vi "Record_to_TDMS.vi"() -> ()   [LabVIEW 2019]
uses:
  SubVIs/TypeDefs/StateRecording.ctl
  <vilib>/DAQmx/read.llb/DAQmx Read (Analog 1D Wfm NChan NSamp).vi
  <vilib>/DAQmx/create/channels.llb/DAQmx Create Channel (AI-Voltage-Basic).vi
  <vilib>/DAQmx/configure/timing.llb/DAQmx Timing (Sample Clock).vi
  <vilib>/DAQmx/miscellaneous.llb/DAQmx Fill In Error Info.vi
  <vilib>/measure/madcrms.llb/Basic Averaged DC-RMS for 1 Chan.vi
  <vilib>/express/express analysis/Spectral/Block/exnSpectralBlock spectral measurements RMS poly.vi
  <vilib>/express/express analysis/Spectral/Block/exnSpectralBlock spectral measurements RMS WFM.vi
  <vilib>/express/express analysis/Spectral/XNode/ExpressSpectralMeasurementsBlockNode.xnode
  <vilib>/measure/NI_MAPro.lvlib
panel:
  out "Elapsed Time (s)":dbl
  in  "stop":bool
  in  "Pause time [s]":dbl=15.0 caption="Time Target (s)"
  out "State":string
  in  "Record":bool
  out "Waveform":waveform(dbl)[](graph)
  out "Spectrum":cluster{"f0":dbl, "df":dbl, "magnitude":dbl[]}(graph)
  in  "sample rate":dbl=10000.0 format="%#_13g"
  in  "samples per channel":i32=10000
  in  "Filename":string
  in  "Recording time [s]":dbl=15.0 caption="Time Target (s)"
  in  "Number of recordings":i32
  in  "Recording directory":path
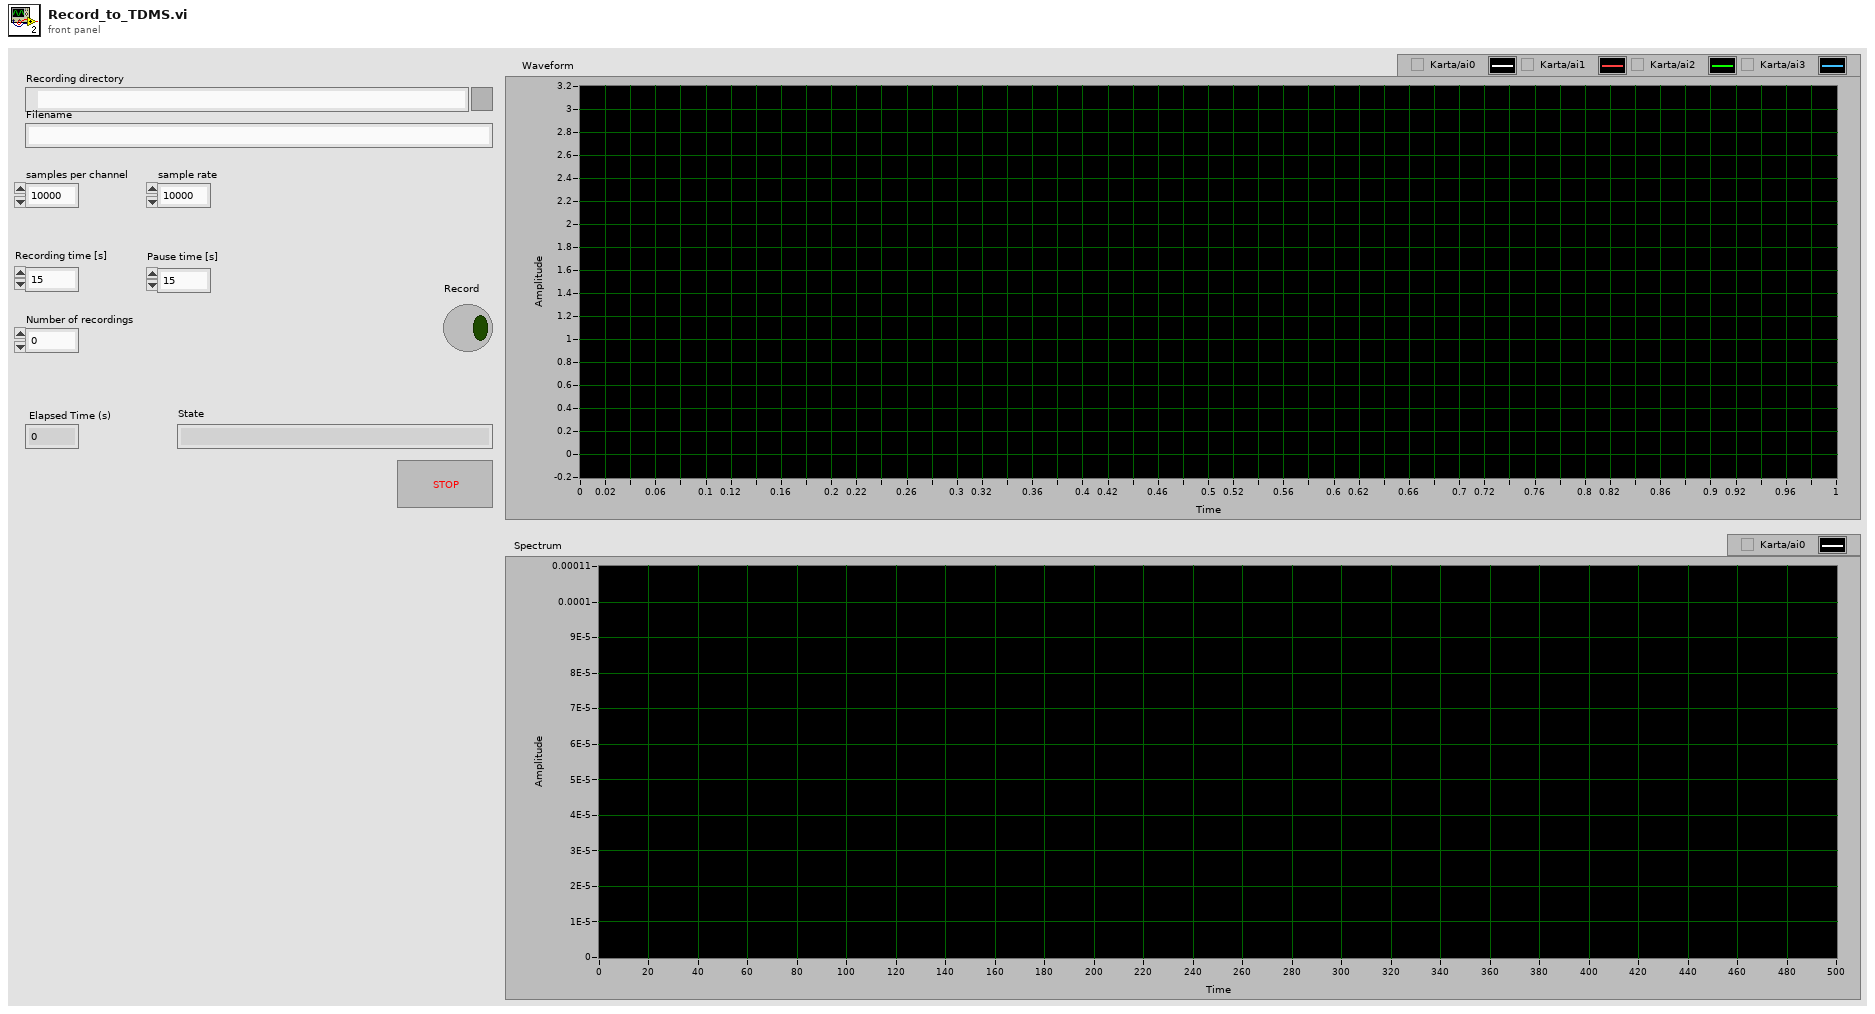
[diagram p1: front panel]
types:
  T1 = typedef "StateRecording.ctl" = enum16{"IDLE", "RECORDING", "PAUSE"}
  T2 = enum16{"open", "open or create", "create or replace", "create", "open (read-only)"}
  T3 = cluster{"averaging mode":u16, "weighting mode":u16, "number of averages":u32}
  T4 = cluster{"dB On (F)":bool, "unwrap phase (F)":bool, "convert to degree (F)":bool}
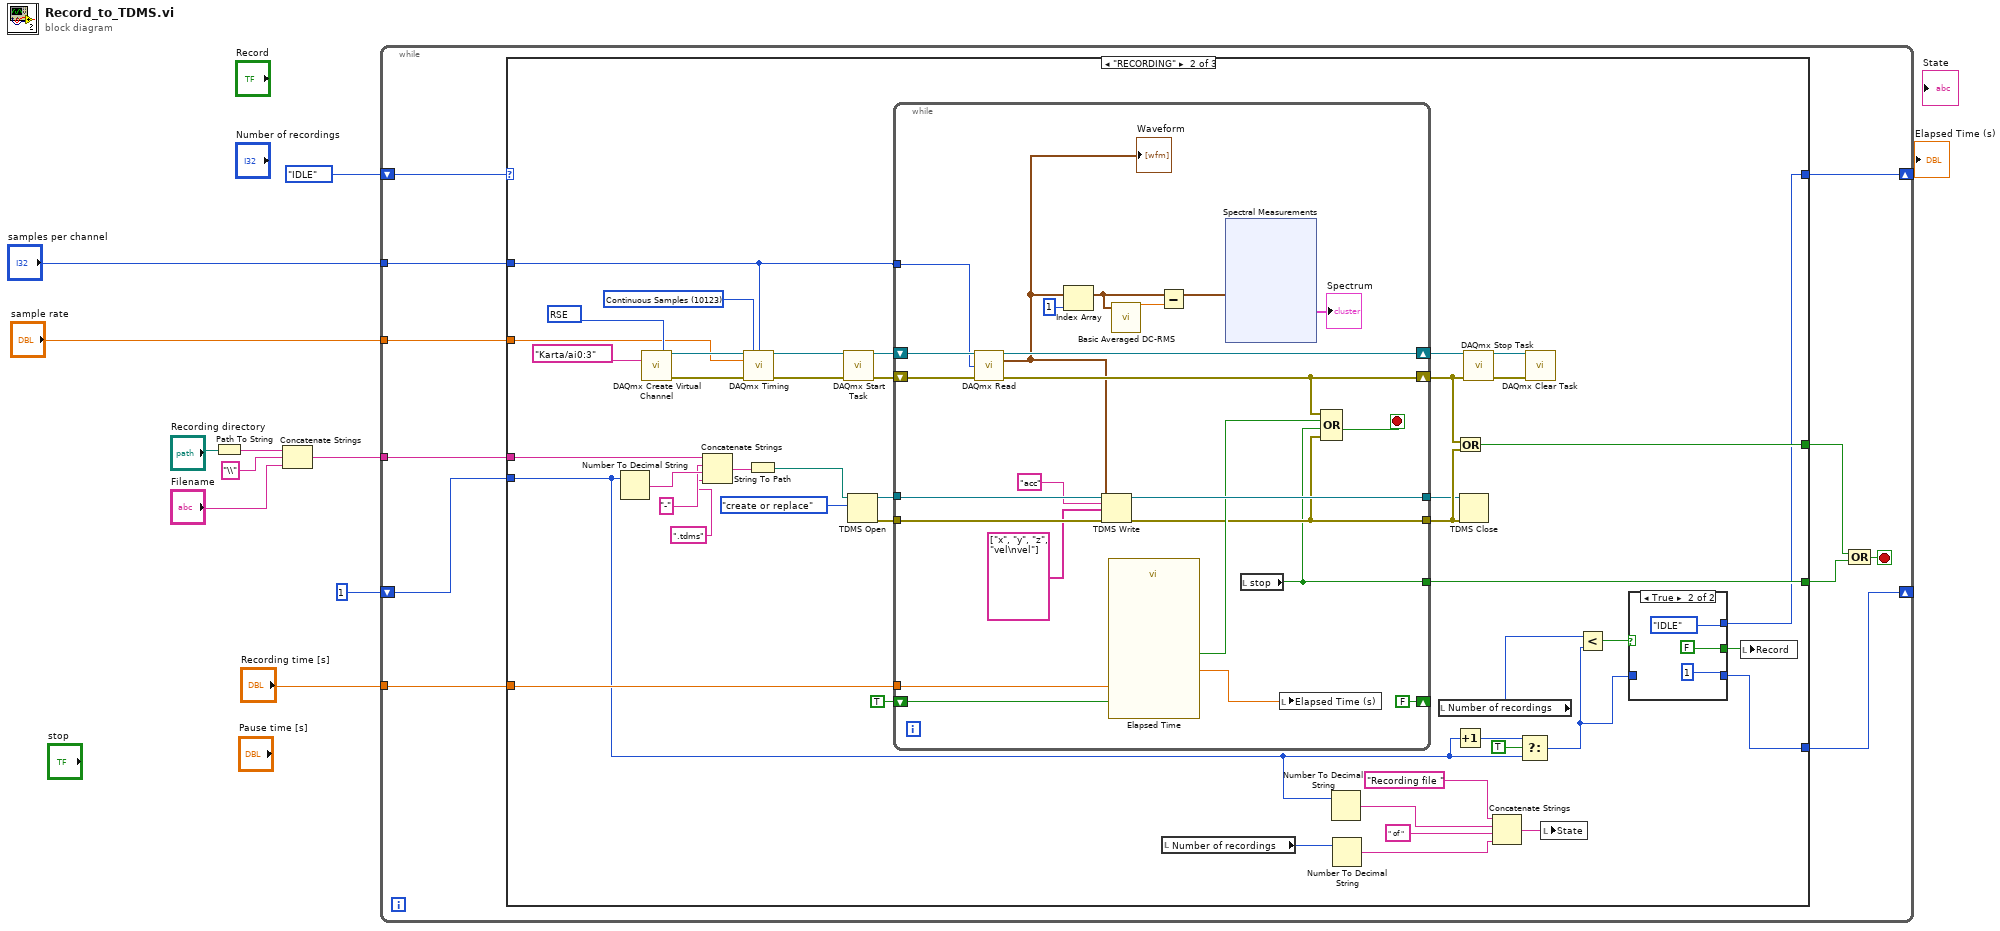
[diagram p0: block diagram]
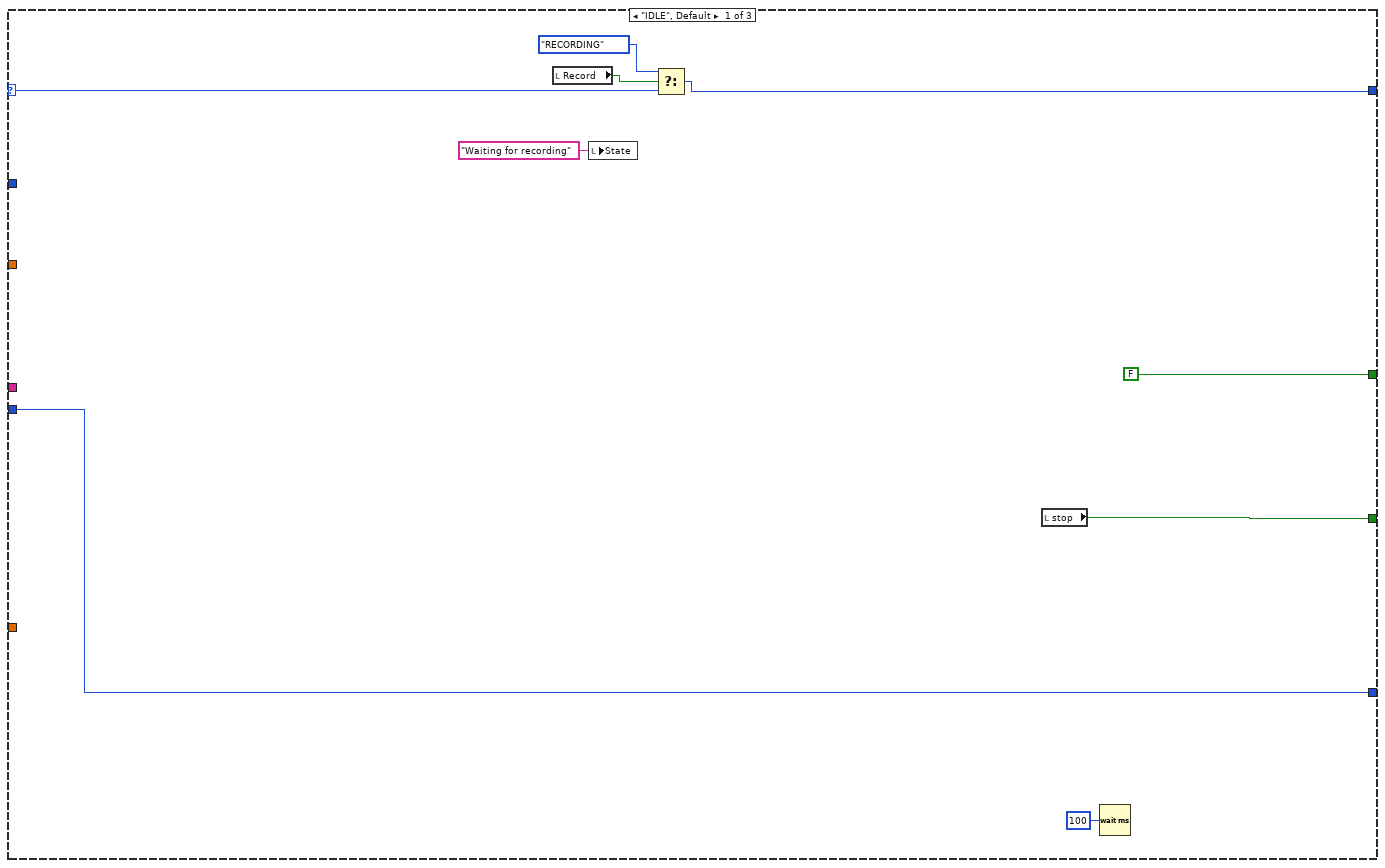
[diagram p2: hidden frame]
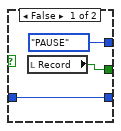
[diagram p3: hidden frame]
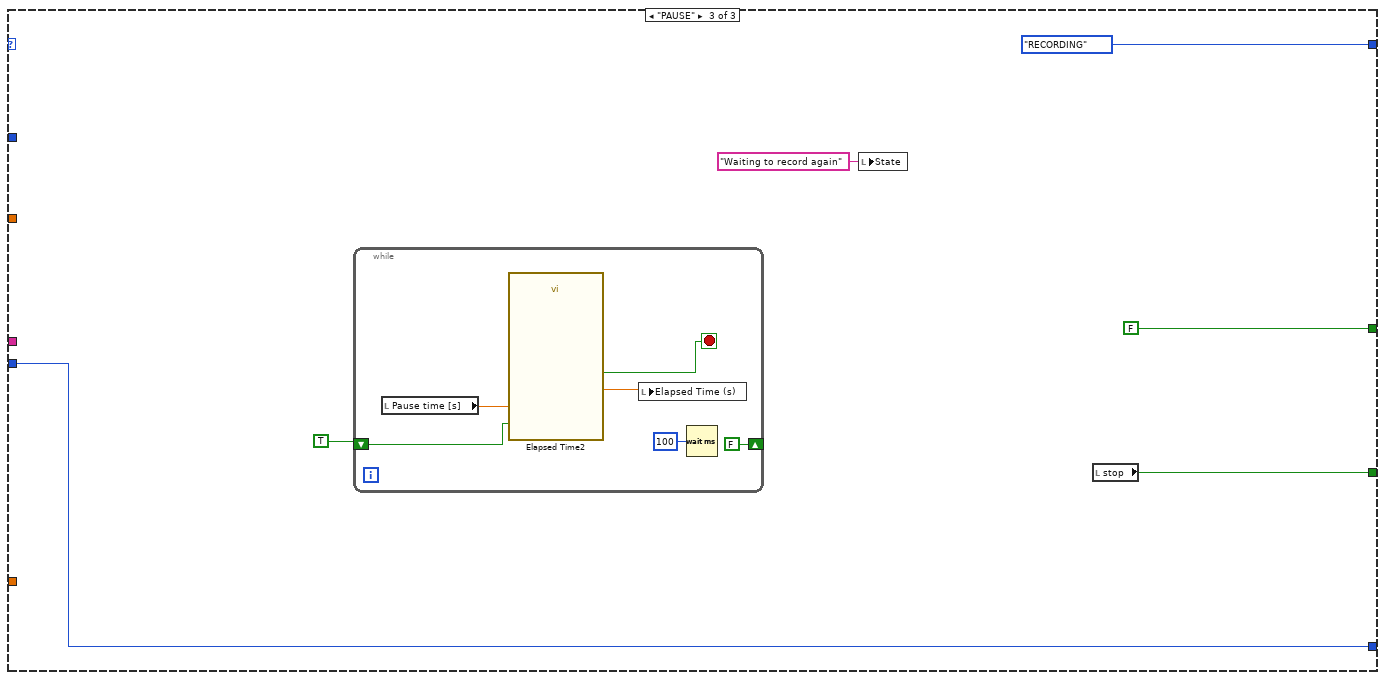
[diagram p4: hidden frame]
diagram:
  n1 = Path To String(path="Recording directory") -> (string=w9:string)
  n2 = Concatenate Strings(w9, "\\" ("string"), "Filename") -> (w6:string)
  n3 = while {
    tunnel: w6 -> [w21]
    tunnel: "Recording time [s]" -> [w20]
    shift-right: [w16] -> _
    shift-left: 1 -> [w19]
    shift-right: [w17] -> _
    shift-left: StateRecording."IDLE" -> [w18]
    tunnel: "samples per channel" -> [w12]
    tunnel: "sample rate" -> [w11]
    stop <- w15 stop-if-true
    n4 = case shown="\"RECORDING\"" w18 {
      selector: w18 -> [w28 _ _]
      tunnel: w21 -> [_ w64 _]
      tunnel: w20 -> [_ w63 _]
      tunnel: w19 -> [w29 w55 w120]
      tunnel: [w29 w31 w120] -> w16
      tunnel: [w30 w50 w121] -> w14
      tunnel: [w25 w34 StateRecording."RECORDING"] -> w17
      tunnel: [FALSE w49 FALSE] -> w13
      tunnel: w12 -> [_ w43 _]
      tunnel: w11 -> [_ w42 _]
      frame "IDLE", Default {
        n5 = local read "Record"() -> (w27:bool)
        n6 = local write "State"("Waiting for recording" ("State")) -> ()
        n7 = Select(t=StateRecording."RECORDING", s=w27, f=w28) -> (s? t:f=w25:T1)
        n8 = local read "stop"() -> (w30:bool)
        n9 = Wait (ms)(milliseconds to wait=u32 100) -> ()  [unwired: 1 out]
      }
      frame "RECORDING" {
        w45 = 10083 items=["Default"=-1, "RSE"=10083, "NRSE"=10078, "Differential"=10106, "Pseudodifferential"=12529] ("input terminal configuration")
        w46 = 10123 items=["Finite Samples"=10178, "Continuous Samples"=10123, "Hardware Timed Single Point"=12522] ("sample mode")
        n10 = Number To Decimal String(number=w55) -> (decimal integer string=w73:string)  [unwired: 1 in]
        n11 = call-poly <vilib>:"DAQmx Create Virtual Channel.vi"("input terminal configuration"=w45, "physical channels"=tag "Karta/ai0:3") -> ("task out"=w47:refnum<k21>, "error out"=w48:errorcluster)  [unwired: 12 in]
        n12 = Concatenate Strings(w64, "-" ("string"), w73, ".tdms" ("string")) -> (w74:string)
        n13 = call-poly <vilib>:"DAQmx Timing.vi"("task/channels in"=w47, "sample mode"=w46, "samples per channel"=w43, "rate"=w42, "error in"=w48) -> ("task out"=w41:refnum<k21>, "error out"=w40:errorcluster)  [unwired: 9 in]
        n14 = String To Path(string=w74) -> (path=w75:path)
        n15 = call <vilib>:"DAQmx Start Task.vi"("task/channels in"=w41, "error in"=w40) -> ("task out"=w68:refnum<k21>, "error out"=w69:errorcluster)  [unwired: 12 in]
        n16 = TDMS Open(10:T2."create or replace" ("operation (0:open)"), 11:w75) -> (0:w72:errorcluster, 3:w71:refnum<k34>)  [unwired: 5 in]
        n17 = while {
          tunnel: w71 -> [w101]
          tunnel: w72 -> [w102]
          tunnel: [w100] -> w60
          tunnel: [w92] -> w62
          shift-right: [w103] -> w70
          shift-left: w68 -> [w105]
          shift-right: [w98] -> w61
          shift-left: w69 -> [w104]
          tunnel: w63 -> [w97]
          tunnel: w43 -> [w96]
          tunnel: [w85] -> w50
          shift-right: [FALSE] -> _
          shift-left: TRUE -> [w83]
          stop <- w99 stop-if-true
          n18 = call-poly <vilib>:"DAQmx Read.vi"("task/channels in"=w105, "number of samples per channel"=w96, "error in"=w104) -> ("task out"=w103:refnum<k21>, "data"=w90:waveform(dbl)[], "error out"=w98:errorcluster)  [unwired: 10 in]
          "Waveform" <- w90
          n19 = Index Array(array=w90, index=1) -> (element=w88:waveform(dbl))
          n20 = TDMS Write(0:w101, 5:"acc" ("group name in (Untitled)"), 7:string[] ["x", "y", "z", "vel\nvel"] ("channel name(s) in (Untitled)"), 9:w90, 11:w102) -> (4:w100:refnum<k34>, 15:w92:errorcluster)  [unwired: 1 in, 2 out]
          n21 = call "Elapsed Time"("Time Target (s)"=w97, "Reset"=w83) -> ("Elapsed Time (s)"=w84:dbl, "Time has Elapsed"=w95:bool)  [unwired: 10 in, 6 out]
          n22 = call-poly <vilib>:"Basic Averaged DC-RMS.vi"("signal in"=w88) -> ("DC value"=w86:dbl)  [unwired: 7 in, 3 out]
          n23 = Subtract(x=w88, y=w86) -> (x-y=w87:waveform(dbl))
          n24 = xnode "Spectral Measurements"("Signals"=w87) -> ("FFT - (RMS)"=→"Spectrum":cluster{"f0":dbl, "df":dbl, "magnitude":dbl[]})  [unwired: 1 in, 2 out]
          n25 = local read "stop"() -> (w85:bool)
          n26 = local write "Elapsed Time (s)"(w84) -> ()
          n27 = Compound Arithmetic op=OR(w98, w95, w85, w92) -> (w99:bool)
        }
        n28 = local read "Number of recordings"() -> (w52:i32)
        n29 = Number To Decimal String(number=w55) -> (decimal integer string=w54:string)  [unwired: 1 in]
        n30 = Number To Decimal String(number=w52) -> (decimal integer string=w53:string)  [unwired: 1 in]
        n31 = local read "Number of recordings"() -> (w36:i32)
        n32 = Increment(x=w55) -> (x+1=w59:i32)
        n33 = Or(x=w61, y=w62) -> (x .or. y?=w49:bool)
        n34 = TDMS Close(8:w62, 11:w60) -> ()  [unwired: 2 out]
        n35 = call <vilib>:"DAQmx Stop Task.vi"("task/channels in"=w70, "error in"=w61) -> ("task out"=w39:refnum<k21>, "error out"=w38:errorcluster)  [unwired: 12 in]
        n36 = Concatenate Strings("Recording file " ("State"), w54, " of " ("string"), w53) -> (w58:string)
        n37 = Select(t=w59, s=TRUE, f=w55) -> (s? t:f=w32:i32)
        n38 = call <vilib>:"DAQmx Clear Task.vi"("task in"=w39, "error in"=w38) -> ()  [unwired: 13 in, 1 out]
        n39 = local write "State"(w58) -> ()
        n40 = Less?(x=w36, y=w32) -> (x < y?=w35:bool)
        n41 = case shown="True" w35 {
          tunnel: w32 -> [w78 _]
          tunnel: [w78 1] -> w31
          tunnel: [StateRecording."PAUSE" StateRecording."IDLE"] -> w34
          tunnel: [w76 FALSE ("t")] -> w33
          frame False {
            n42 = local read "Record"() -> (w76:bool)
          }
          frame True {
          }
        }
        n43 = local write "Record"(w33) -> ()
      }
      frame "PAUSE" {
        n44 = while {
          shift-right: [FALSE] -> _
          shift-left: TRUE -> [w123]
          stop <- w124 stop-if-true
          n45 = local read "Pause time [s]"() -> (w126:dbl)
          n46 = call "Elapsed Time2"("Time Target (s)"=w126, "Reset"=w123) -> ("Elapsed Time (s)"=w127:dbl, "Time has Elapsed"=w124:bool)  [unwired: 10 in, 6 out]
          n47 = local write "Elapsed Time (s)"(w127) -> ()
          n48 = Wait (ms)(milliseconds to wait=u32 100) -> ()  [unwired: 1 out]
        }
        n49 = local write "State"("Waiting to record again" ("State")) -> ()
        n50 = local read "stop"() -> (w121:bool)
      }
    }
    n51 = Compound Arithmetic op=OR(w13, w14) -> (w15:bool)
  }
